vi "Write Outgoing Bytes.vi"(8 "error in (no error)":errorcluster, 10 "Bytes":u8[](array[numeric]) format="%08b", 11 "TCPConnection in":refnum<class "TCPConnection.lvclass">) -> (0 "error out":errorcluster, 3 "TCPConnection out":refnum<class "TCPConnection.lvclass">)   [LabVIEW 2013, in "MQTT Server.lvlib" / "TCPConnection.lvclass"]
uses:
  TCPConnection.lvclass
  TCPConnection.lvclass/TCPConnection.ctl
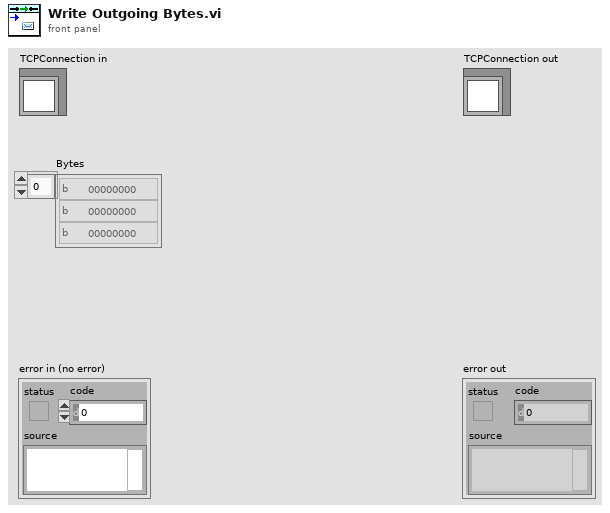
[diagram p1: front panel]
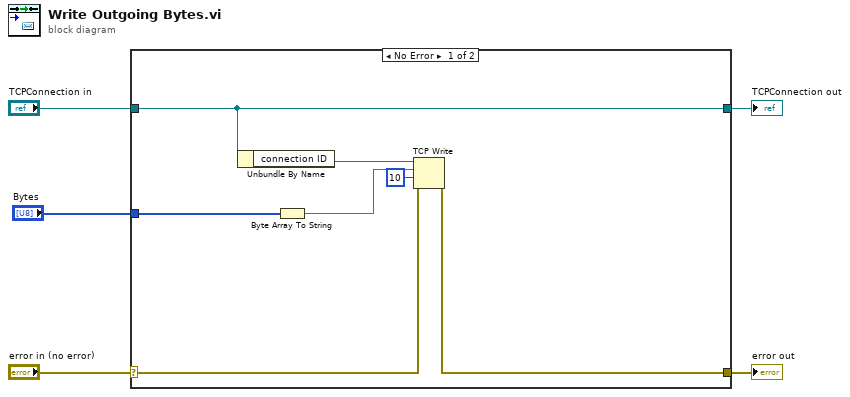
[diagram p0: block diagram]
diagram:
  n1 = case shown="No Error" "error in (no error)" {
    selector: "error in (no error)" -> [w7 w14]
    tunnel: [w6 w14] -> w4
    tunnel: [w12 w13] -> w2
    tunnel: "TCPConnection in" -> [w12 w13]
    tunnel: "Bytes" -> [w10 _]
    frame No Error {
      n2 = Unbundle By Name(w12) -> ("connection ID"=w11:refnum<k5>)
      n3 = Byte Array To String(unsigned byte array=w10) -> (string=w9:string)
      n4 = TCP Write(connection ID=w11, data in=w9, error in (no error)=w7, 9:10 ("timeout ms (25000)")) -> (error out=w6:errorcluster)  [unwired: 2 out]
    }
    frame Error {
    }
  }
  "error out" <- w4
  "TCPConnection out" <- w2
